vi "Test - New VI Object.vi"() -> ()   [LabVIEW 2015]
doc: "This VI is used by the New VI Object Location Argument.vi example."
panel:
  out "read buffer":string
  in  "VISA resource name":refnum<visa-resource-name>
  in  "Anchor 4":dbl
  in  "Anchor 3":dbl
  out "Cluster":T1
  # "<------------ Point 100, 20"
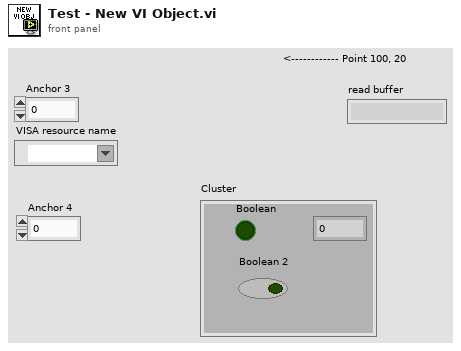
[diagram p1: front panel]
types:
  T1 = cluster{"Boolean":bool, "Boolean 2":bool, "Numeric":dbl}
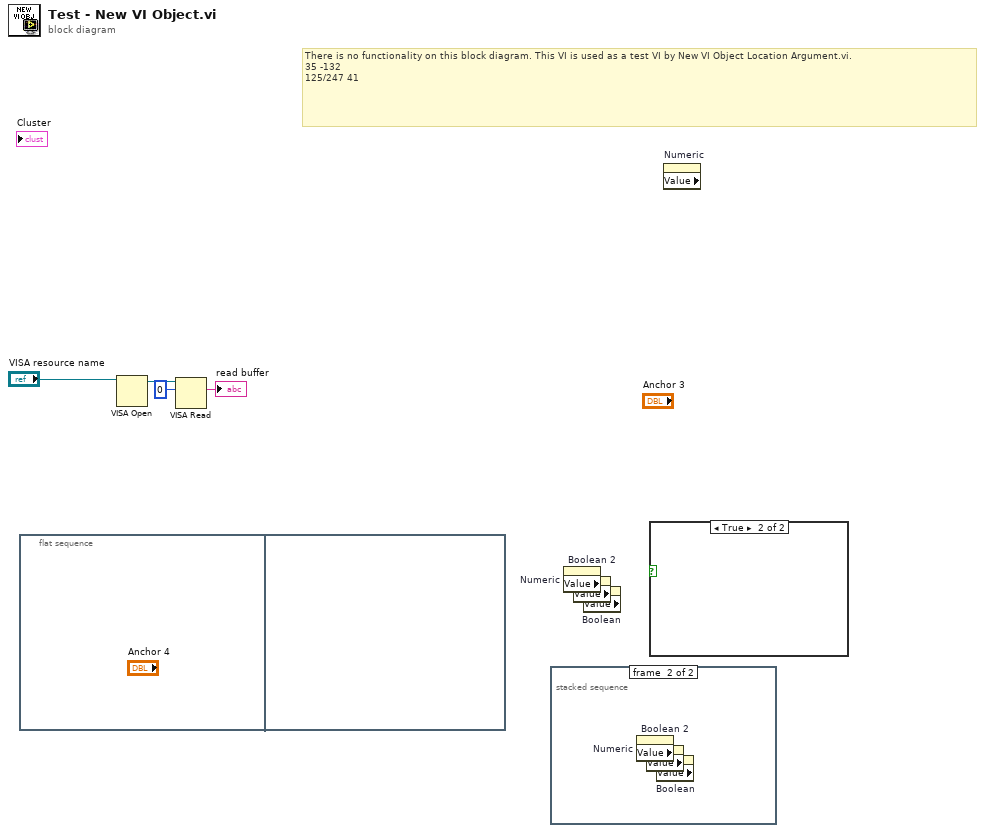
[diagram p0: block diagram]
diagram:
  # "There is no functionality on this block diagram. This VI is used as a test VI by New VI Object Location Argument.vi.\n35 -132\n125/247 41"
  n1 = flat-sequence {
    frame #0 {
    }
    frame #1 {
    }
  }
  n2 = VISA Open(VISA resource name="VISA resource name") -> (VISA resource name=w4:refnum<visa-resource-name>)  [unwired: 4 in, 1 out]
  n3 = VISA Read(VISA resource name=w4, byte count=u32 0) -> (read buffer=→"read buffer":string)  [unwired: 1 in, 3 out]
  n4 = stacked-sequence {
    frame #0 {
    }
    frame #1 {
      n5 = property on="Numeric" class="DigNum (strict)" props=["Value"]() -> ()  [unwired: 2 in, 3 out]
      n6 = property on="Boolean 2" class="Bool (strict)" props=["Value"]() -> ()  [unwired: 2 in, 3 out]
      n7 = property on="Boolean" class="Bool (strict)" props=["Value"]() -> ()  [unwired: 2 in, 3 out]
    }
  }
  n8 = property on="Numeric" class="DigNum (strict)" props=["Value"]() -> ()  [unwired: 2 in, 3 out]
  n9 = property on="Boolean 2" class="Bool (strict)" props=["Value"]() -> ()  [unwired: 2 in, 3 out]
  n10 = property on="Boolean" class="Bool (strict)" props=["Value"]() -> ()  [unwired: 2 in, 3 out]
  n11 = case shown="True" {
    selector: _ -> [_ _]
    frame False {
    }
    frame True {
    }
  }
  n12 = property on="Numeric" class="DigNum (strict)" props=["Value"]() -> ()  [unwired: 2 in, 3 out]
